vi "Tx Cyclic Write.vi"(8 "error in (no error)":errorcluster, 10 "Data":dbl[](array[numeric]), 11 "Tx Cyclic In":T1) -> (0 "error out":errorcluster, 3 "Tx Cyclic Out":T1)   [LabVIEW 2020, in "985x Support Addon Engine.lvlib"]
uses:
  985x Support Addon Engine.lvlib
  Types/Cyclic Frame Info.ctl
  Types/Tx Cyclic Session.ctl
  Types/FPGA Refnum.ctl
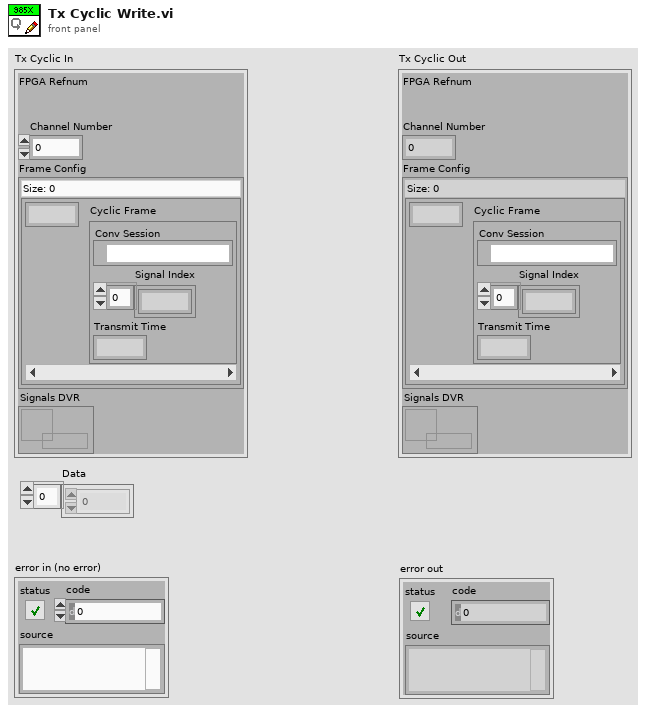
[diagram p1: front panel]
types:
  T1 = typedef "985x Support Addon Engine.lvlib/Tx Cyclic Session.ctl" = cluster{"FPGA Refnum":T2, "Channel Number":u32, "Frame Config":map{u32, T3}, "Signals DVR":refnum<data-value>}
  T2 = typedef "985x Support Addon Engine.lvlib/FPGA Refnum.ctl" = refnum<k20>
  T3 = typedef "985x Support Addon Engine.lvlib/Cyclic Frame Info.ctl" = cluster{"Conv Session":refnum<k21>, "Signal Index":u32[], "Transmit Time":dbl}
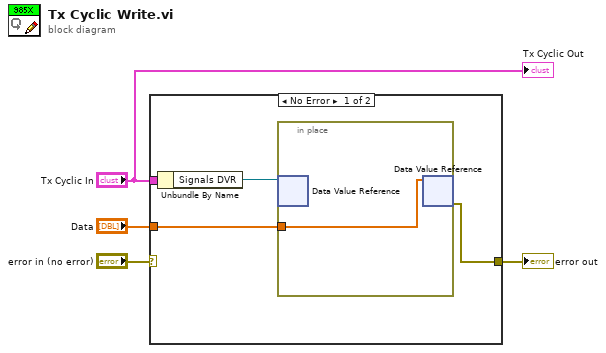
[diagram p0: block diagram]
diagram:
  n1 = case shown="No Error" "error in (no error)" {
    selector: "error in (no error)" -> [_ w10]
    tunnel: "Tx Cyclic In" -> [w8 _]
    tunnel: "Data" -> [w6 _]
    tunnel: [w5 w10] -> w2
    frame No Error {
      n2 = Unbundle By Name(w8) -> ("Signals DVR"=w7:refnum<data-value>)
      n3 = in-place {
        in-place-border: w6 -> [w9]
        n4 = in-place-dvr #1(w7) -> ()  [unwired: 2 out]
        n5 = in-place-dvr #1(w9) -> (w5:errorcluster)  [unwired: 1 out]
      }
    }
    frame Error {
    }
  }
  "error out" <- w2
  "Tx Cyclic Out" <- "Tx Cyclic In"
